vi "SyncVI.vi"(3 "ControlIndicator":T2(array[cluster]), 4 "vi reference":refnum<vi>, 5 "ArrayOfComands":variant) -> (2 "Response":string)   [LabVIEW 2010]
panel:
  out "Temp":string
  out "ArrayOfCommands":T1(array[cluster])
  in  "comand recieved":T3
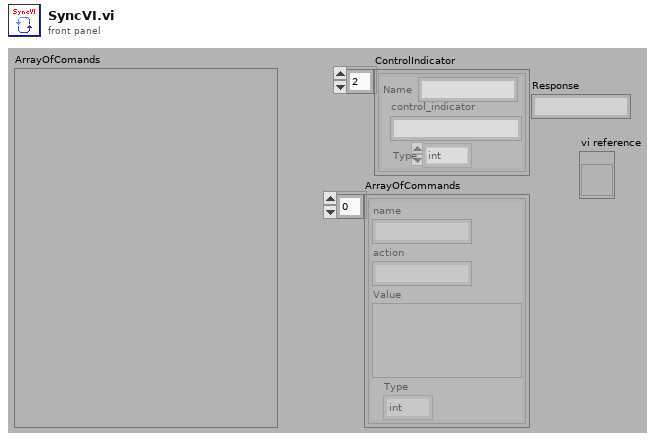
[diagram p1: front panel]
types:
  T1 = cluster{"name":string, "action":string, "Value":variant, "Type":enum16{"int", "boolean", "string", "double", "dateTime", "base64", "struct", "array"}}[]
  T2 = cluster{"Name":string, "control_indicator":string, "Type":enum16{"int", "boolean", "string", "double", "dateTime", "base64", "struct", "array"}}[]
  T3 = cluster{"name":string, "action":string, "Value":variant, "Type":enum16{"int", "boolean", "string", "double", "dateTime", "base64", "struct", "array"}}
  T4 = enum16{"int", "boolean", "string", "double", "dateTime", "base64", "struct", "array"}[]
  T5 = enum16{"int", "boolean", "string", "double", "dateTime", "base64", "struct", "array"}
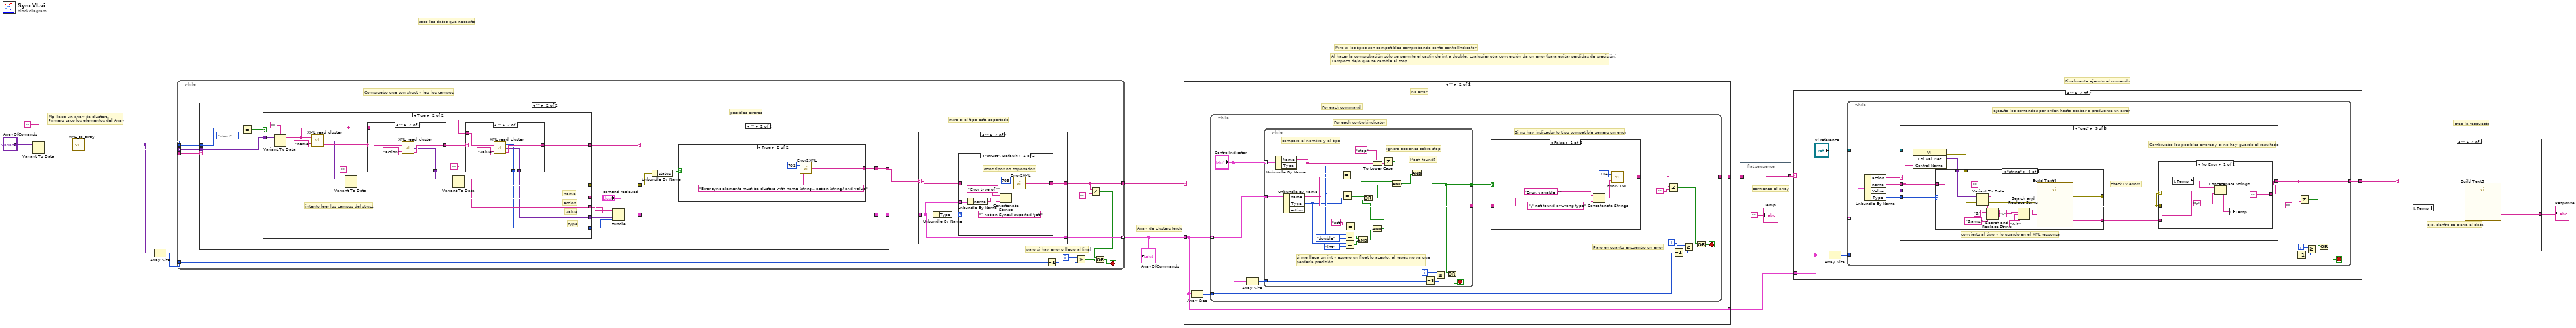
[diagram p0: block diagram]
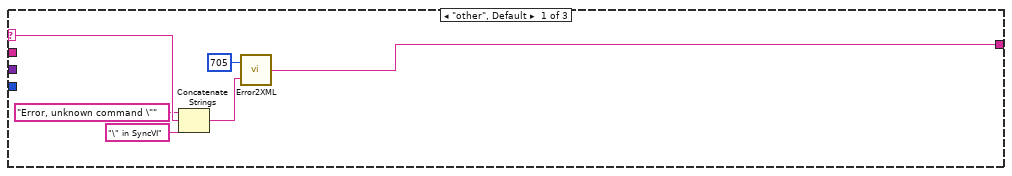
[diagram p4: hidden frame]
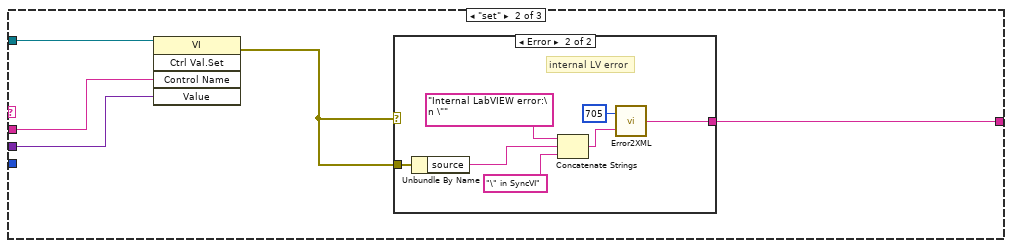
[diagram p5: hidden frame]
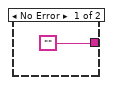
[diagram p6: hidden frame]
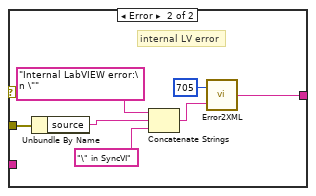
[diagram p7: hidden frame]
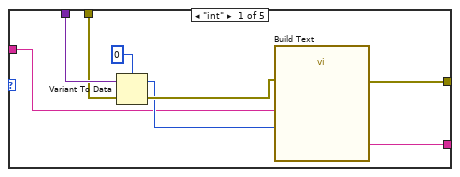
[diagram p8: hidden frame]
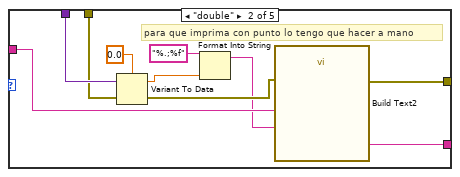
[diagram p9: hidden frame]
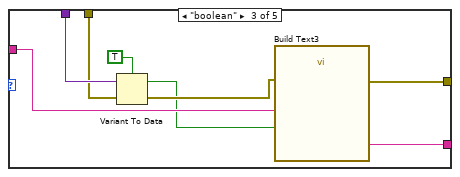
[diagram p10: hidden frame]
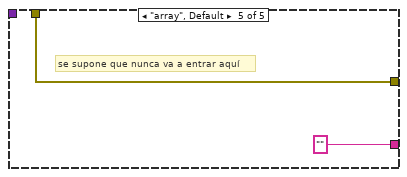
[diagram p11: hidden frame]
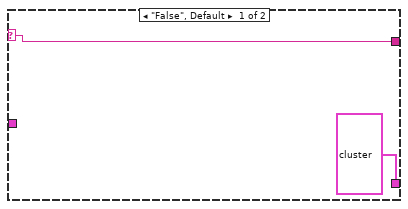
[diagram p12: hidden frame]
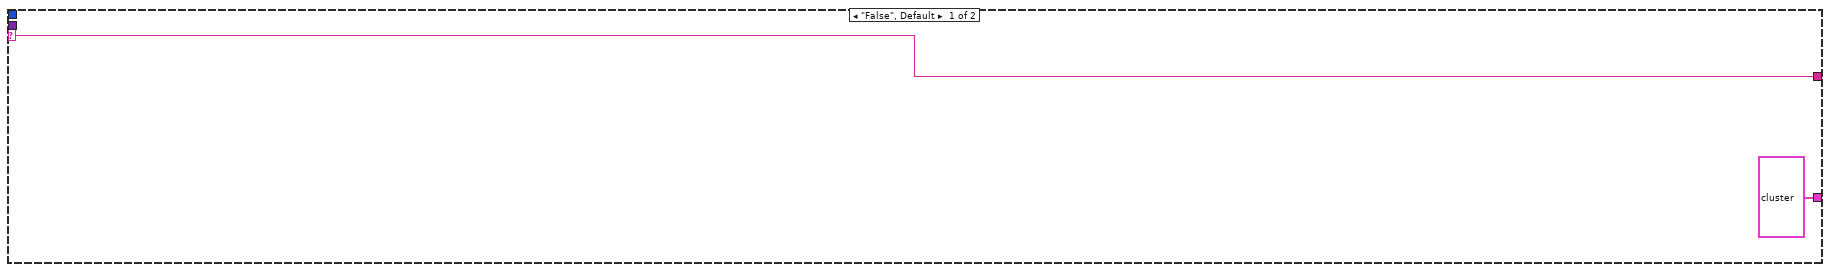
[diagram p14: hidden frame]
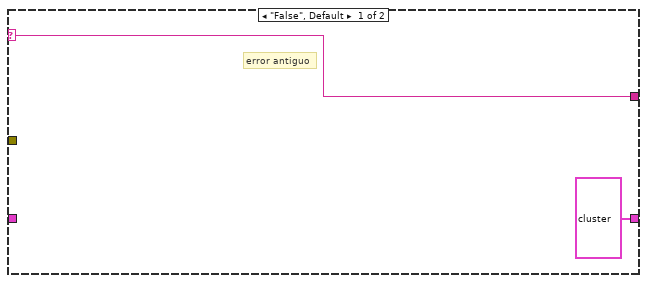
[diagram p15: hidden frame]
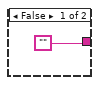
[diagram p16: hidden frame]
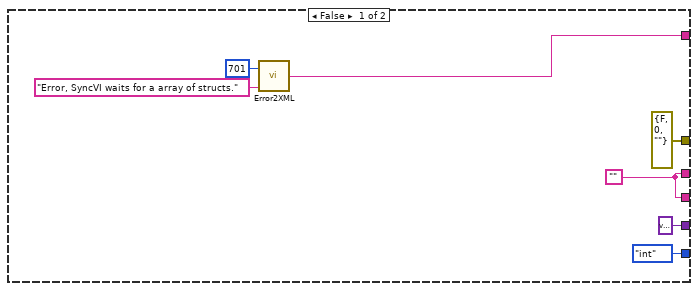
[diagram p17: hidden frame]
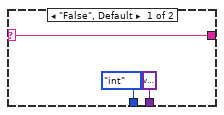
[diagram p18: hidden frame]
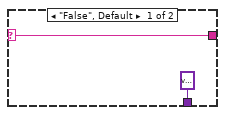
[diagram p19: hidden frame]
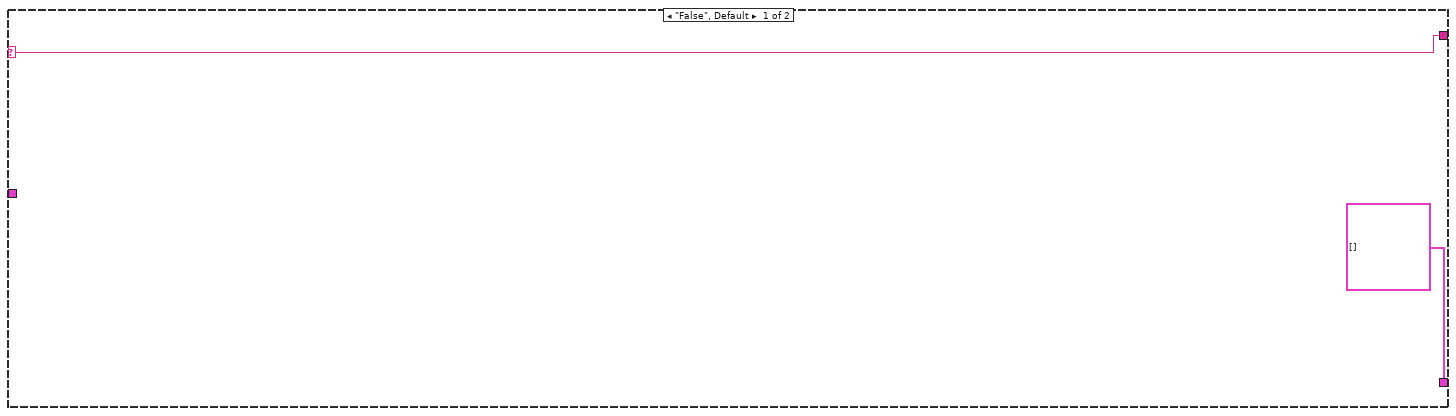
[diagram p20: hidden frame]
diagram:
  # "Al hacer la comprobación sólo se permite el castin de int a double, cualquier otra conversión da un error (para evitar perdidas de precisión)\nTampoco dejo que se cambie el stop"
  # "creo la respuesta"
  # "Finalmente ejecuto el comando"
  # "Miro si los tipos son compatibles comprobando conta controlIndicator"
  # "Array de clusters leido"
  # "saco los datos que necesito"
  # "Me llega un array de clusters.\nPrimero saco los elementos del Array"
  n1 = Variant To Data(Variant="ArrayOfComands", type="") -> (data=w12:string)  [unwired: 1 in, 1 out]
  n2 = call "XML_to_array.vi"("XML"=w12) -> ("ParsingErrors"=w11:string, "Values"=w9:variant[], "Types"=w10:T4)
  n3 = Array Size(array=w9) -> (size(s)=w7:i32)
  n4 = while {
    tunnel: w11 -> [w28]
    tunnel: w10 -> [w27] mode=indexing
    tunnel: w9 -> [w26] mode=indexing
    tunnel: [w17] -> w8
    tunnel: [w23] -> w6 mode=indexing
    tunnel: w7 -> [w21]
    i -> [w22]
    stop <- w19 stop-if-true
    # "paro si hay error o llego al final"
    # "miro si el tipo está soportado"
    # "Compruebo que son struct y leo los campos"
    n5 = case shown="\"\"" w28 {
      selector: w28 -> [w44 _]
      tunnel: w27 -> [_ w58]
      tunnel: w26 -> [_ w55]
      tunnel: [w44 w46] -> w24
      tunnel: [T3 {"name"="", "action"="", "Value"=variant, "Type"=enum."int"} ("comand recieved") w45] -> w25
      frame "False", Default {
      }
      frame "" {
        # "posibles errores"
        n6 = Equal?(x=w58, y=T5."struct") -> (x = y?=w56:bool)
        n7 = case shown="True" w56 {
          tunnel: w55 -> [_ w92]
          tunnel: [w73 w82] -> w54
          tunnel: [errorcluster {"status"=FALSE, "code"=0, "source"=""} ("error out") w79] -> w53
          tunnel: [w71 w81] -> w52
          tunnel: [w71 w80] -> w51
          tunnel: [T5."int" ("Type") w78] -> w49
          tunnel: [variant ("Value") w77] -> w50
          frame False {
            w71 = ""
            n8 = call "Error2XML.vi"("FailDescriptor"="Error, SyncVI waits for a array of structs.", "FailID"=701) -> ("ErrorXML"=w73:string)
          }
          frame True {
            # "type"
            # "value"
            # "action"
            # "name"
            # "intento leer los campos del struct"
            n9 = Variant To Data(Variant=w92, type="") -> (data=w76:string)  [unwired: 1 in, 1 out]
            n10 = call "XML_read_cluster.vi"("Name"="name", "XML"=w76) -> ("ParsingErrors"=w89:string, "Value"=w87:variant)  [unwired: 1 out]
            n11 = Variant To Data(Variant=w87, type="") -> (error out=w85:errorcluster, data=w81:string)  [unwired: 1 in]
            n12 = case shown="\"\"" w89 {
              selector: w89 -> [w102 _]
              tunnel: [w102 w105] -> w88
              tunnel: [variant ("Value") w104] -> w84
              tunnel: w76 -> [_ w103]
              frame "False", Default {
              }
              frame "" {
                n13 = call "XML_read_cluster.vi"("Name"="action", "XML"=w103) -> ("ParsingErrors"=w105:string, "Value"=w104:variant)  [unwired: 1 out]
              }
            }
            n14 = Variant To Data(error in=w85, Variant=w84, type="") -> (error out=w79:errorcluster, data=w80:string)
            n15 = case shown="\"\"" w88 {
              selector: w88 -> [w95 _]
              tunnel: [w95 w100] -> w82
              tunnel: [variant ("Value") w98] -> w77
              tunnel: [T5."int" ("Type") w97] -> w78
              tunnel: w76 -> [_ w96]
              frame "False", Default {
              }
              frame "" {
                n16 = call "XML_read_cluster.vi"("Name"="value", "XML"=w96) -> ("ParsingErrors"=w100:string, "Value"=w98:variant, "Type"=w97:T5)
              }
            }
          }
        }
        n17 = Bundle(cluster="comand recieved", "name"=w52, "action"=w51, "Value"=w50, "Type"=w49) -> (w47:T3)
        n18 = case shown="\"\"" w54 {
          selector: w54 -> [w60 _]
          tunnel: [w60 w64] -> w46
          tunnel: w53 -> [_ w63]
          tunnel: [T3 {"name"="", "action"="", "Value"=variant, "Type"=enum."int"} ("comand recieved") w61] -> w45
          tunnel: w47 -> [_ w61]
          frame "False", Default {
            # "error antiguo"
          }
          frame "" {
            n19 = Unbundle By Name(w63) -> ("status"=w62:bool)
            n20 = case shown="True" w62 {
              tunnel: ["" w66] -> w64
              frame False {
              }
              frame True {
                n21 = call "Error2XML.vi"("FailDescriptor"="Error sync elements must be clusters with name (string), action (string) and value", "FailID"=702) -> ("ErrorXML"=w66:string)
              }
            }
          }
        }
      }
    }
    n22 = case shown="\"\"" w24 {
      selector: w24 -> [w30 w32]
      tunnel: w25 -> [_ w31]
      tunnel: [w30 w33] -> w17
      tunnel: [T3 {"name"="", "action"="", "Value"=variant, "Type"=enum."int"} ("comand recieved") w31] -> w23
      frame "False", Default {
      }
      frame "" {
        n23 = Unbundle By Name(w31) -> ("Type"=w34:T5)
        n24 = case shown="\"struct\", Default" w34 {
          tunnel: w31 -> [w39 _]
          tunnel: [w35 w42] -> w33
          tunnel: w32 -> [_ w42]
          frame "struct", Default {
            # "otros tipos no soportados"
            n25 = Unbundle By Name(w39) -> ("name"=w38:string)
            n26 = Concatenate Strings("Error type of “" ("string"), w38, "” not on SyncVI suported (jet)" ("string")) -> (w40:string)
            n27 = call "Error2XML.vi"("FailDescriptor"=w40, "FailID"=703) -> ("ErrorXML"=w35:string)
          }
          frame "int".."double" {
            # "todo ok"
          }
        }
      }
    }
    n28 = Decrement(x=w21) -> (x-1=w20:i32)
    n29 = Greater Or Equal?(x=w22, y=w20) -> (x >= y?=w18:bool)
    n30 = Not Equal?(x=w17, y="") -> (x != y?=w15:bool)
    n31 = Or(x=w15, y=w18) -> (x .or. y?=w19:bool)
  }
  "ArrayOfCommands" <- w6
  n32 = case shown="\"\"" w8 {
    selector: w8 -> [w108 _]
    tunnel: w6 -> [_ w109]
    tunnel: [w108 w110] -> w4
    tunnel: [T1 [] w109] -> w3
    frame "False", Default {
    }
    frame "" {
      # "no error"
      # "For each command"
      n33 = Array Size(array=w109) -> (size(s)=w111:i32)
      n34 = while {
        tunnel: w109 -> [w119] mode=indexing
        tunnel: w111 -> [w123]
        tunnel: [w114] -> w110
        i -> [w122]
        stop <- w121 stop-if-true
        # "Paro en cuanto encuentro un error"
        # "Si no hay indicador to tipo compatible genero un error"
        # "For each control/indicator"
        n35 = Array Size(array="ControlIndicator") -> (size(s)=w117:i32)
        n36 = while {
          tunnel: "ControlIndicator" -> [w158] mode=indexing
          tunnel: w119 -> [w159]
          tunnel: w117 -> [w155]
          tunnel: [w145] -> w116
          tunnel: [w151] -> w115
          i -> [w154]
          stop <- w153 stop-if-true
          # "si me llega un int y espero un float lo acepto, al revés no ya que \nperdería precisión"
          # "ignoro acciones sobre stop"
          # "Mach found?"
          # "comparo el nombre y el tipo"
          n37 = Unbundle By Name(w158) -> ("Name"=w148:string, "Type"=w142:T5)
          n38 = Unbundle By Name(w159) -> ("name"=w151:string, "Type"=w140:T5, "action"=w136:string)
          n39 = Equal?(x=w148, y=w151) -> (x = y?=w157:bool)
          n40 = Equal?(x=w142, y=w140) -> (x = y?=w144:bool)
          n41 = Equal?(x=w142, y=T5."double") -> (x = y?=w137:bool)
          n42 = Equal?(x=w140, y=T5."int") -> (x = y?=w138:bool)
          n43 = Equal?(x="set", y=w136) -> (x = y?=w132:bool)
          n44 = And(x=w137, y=w138) -> (x .and. y?=w134:bool)
          n45 = And(x=w132, y=w134) -> (x .and. y?=w133:bool)
          n46 = Or(x=w144, y=w133) -> (x .or. y?=w143:bool)
          n47 = To Lower Case(string=w148) -> (all lower case string=w149:string)
          n48 = Not Equal?(x="stop" ("y"), y=w149) -> (x != y?=w147:bool)
          n49 = And(x=w157, y=w143) -> (x .and. y?=w146:bool)
          n50 = And(x=w147, y=w146) -> (x .and. y?=w145:bool)
          n51 = Decrement(x=w155) -> (x-1=w156:i32)
          n52 = Greater Or Equal?(x=w154, y=w156) -> (x >= y?=w152:bool)
          n53 = Or(x=w145, y=w152) -> (x .or. y?=w153:bool)
        }
        n54 = case shown="False" w116 {
          tunnel: w115 -> [w129 _]
          tunnel: [w125 ""] -> w114
          frame False {
            n55 = Concatenate Strings("Error: variable \"", w129, "\" not found or wrong type") -> (w126:string)
            n56 = call "Error2XML.vi"("FailDescriptor"=w126, "FailID"=704) -> ("ErrorXML"=w125:string)
          }
          frame True {
            # "OK"
          }
        }
        n57 = Not Equal?(x=w114, y="") -> (x != y?=w112:bool)
        n58 = Decrement(x=w123) -> (x-1=w124:i32)
        n59 = Greater Or Equal?(x=w122, y=w124) -> (x >= y?=w120:bool)
        n60 = Or(x=w112, y=w120) -> (x .or. y?=w121:bool)
      }
    }
  }
  n61 = flat-sequence {
    tunnel: [w161] -> w5
    tunnel: w4 -> [w161]
    frame #0 {
      # "comienzo el array"
      "Temp" <- ""
    }
  }
  n62 = case shown="\"\"" w5 {
    selector: w5 -> [w162 _]
    tunnel: w3 -> [_ w165]
    tunnel: [w162 w163] -> w2
    frame "False", Default {
    }
    frame "" {
      n63 = Array Size(array=w165) -> (size(s)=w164:i32)
      n64 = while {
        tunnel: "vi reference" -> [w172]
        tunnel: w165 -> [w176] mode=indexing
        tunnel: w164 -> [w177]
        tunnel: [w167] -> w163
        i -> [w168]
        stop <- w178 stop-if-true
        # "ejecuto los comandos por orden hasta acabar o producirse un error"
        n65 = Unbundle By Name(w176) -> ("action"=w175:string, "name"=w174:string, "Value"=w173:variant, "Type"=w171:T5)
        n66 = case shown="\"get\"" w175 {
          selector: w175 -> [w185 _ _]
          tunnel: [w181 w187 w201] -> w167
          tunnel: w174 -> [_ w191 w204]
          tunnel: w173 -> [_ w190 _]
          tunnel: w172 -> [_ w189 w207]
          tunnel: w171 -> [_ _ w206]
          frame "other", Default {
            n67 = Concatenate Strings("Error, unknown command \"" ("string"), w185, "\" in SyncVI" ("string")) -> (w182:string)
            n68 = call "Error2XML.vi"("FailDescriptor"=w182, "FailID"=705) -> ("ErrorXML"=w181:string)
          }
          frame "set" {
            n69 = invoke class="VI" method="Ctrl Val.Set"(reference=w189, "Control Name"=w191, "Value"=w190) -> (error out=w188:errorcluster)  [unwired: 2 in, 4 out]
            n70 = case shown="Error" w188 {
              tunnel: ["" w197] -> w187
              tunnel: w188 -> [_ w194]
              frame No Error {
              }
              frame Error {
                # "internal LV error"
                n71 = Unbundle By Name(w194) -> ("source"=w193:string)
                n72 = Concatenate Strings("Internal LabVIEW error:\n \"" ("string"), w193, "\" in SyncVI" ("string")) -> (w198:string)
                n73 = call "Error2XML.vi"("FailDescriptor"=w198, "FailID"=705) -> ("ErrorXML"=w197:string)
              }
            }
          }
          frame "get" {
            # "Combruebo los posibles errores y si no hay guardo el resultado"
            # "check LV errors"
            # "convierto al tipo y lo guardo en el XML response"
            n74 = invoke class="VI" method="Ctrl Val.Get"(reference=w207, "Control Name"=w204) -> (error out=w203:errorcluster, "Get Control Value Variant"=w205:variant)  [unwired: 2 in, 2 out]
            n75 = case shown="\"string\"" w206 {
              tunnel: w205 -> [w227 w237 w245 w260 _]
              tunnel: [w224 w234 w243 w258 w261] -> w200
              tunnel: w204 -> [w222 w233 w242 w257 _]
              tunnel: [w221 w232 w241 w256 "" ("Result")] -> w202
              tunnel: w203 -> [w220 w231 w238 w246 w261]
              frame "int" {
                n76 = Variant To Data(error in=w220, Variant=w227, type=0) -> (error out=w225:errorcluster, data=w223:i32)
                n77 = call "Build Text"("Name"=w222, "Value"=w223, "error in (no error)"=w225) -> ("Result"=w221:string, "error out"=w224:errorcluster)  [unwired: 11 in]
              }
              frame "double" {
                # "para que imprima con punto lo tengo que hacer a mano"
                n78 = Variant To Data(error in=w231, Variant=w237, type=0.0) -> (error out=w235:errorcluster, data=w229:dbl)
                n79 = Format Into String(format string="%.;%f", w229) -> (resulting string=w228:string)  [unwired: 2 in, 1 out]
                n80 = call "Build Text2"("Name"=w233, "Value"=w228, "error in (no error)"=w235) -> ("Result"=w232:string, "error out"=w234:errorcluster)  [unwired: 11 in]
              }
              frame "boolean" {
                n81 = Variant To Data(error in=w238, Variant=w245, type=TRUE) -> (error out=w244:errorcluster, data=w239:bool)
                n82 = call "Build Text3"("Name"=w242, "Value"=w239, "error in (no error)"=w244) -> ("Result"=w241:string, "error out"=w243:errorcluster)  [unwired: 11 in]
              }
              frame "string" {
                n83 = Variant To Data(error in=w246, Variant=w260, type="") -> (error out=w259:errorcluster, data=w247:string)
                n84 = Search and Replace String(input string=w247, search string="&", replace string="&amp;" ("replace string (\"\")")) -> (result string=w249:string, error out=w250:errorcluster)  [unwired: 5 in, 2 out]
                n85 = Search and Replace String(input string=w249, search string="<", replace string="&lt;" ("replace string (\"\")"), error in=w250) -> (result string=w248:string)  [unwired: 4 in, 3 out]
                n86 = call "Build Text4"("Name"=w257, "Value"=w248, "error in (no error)"=w259) -> ("Result"=w256:string, "error out"=w258:errorcluster)  [unwired: 11 in]
              }
              frame "array", Default {
                # "se supone que nunca va a entrar aquí"
              }
            }
            n87 = case shown="No Error" w200 {
              tunnel: ["" w217] -> w201
              tunnel: w202 -> [w208 _]
              tunnel: w200 -> [_ w213]
              frame No Error {
                n88 = local read "Temp"() -> (w211:string)
                n89 = Concatenate Strings(w211, w208, "\r") -> (w209:string)
                n90 = local write "Temp"(w209) -> ()
              }
              frame Error {
                # "internal LV error"
                n91 = Unbundle By Name(w213) -> ("source"=w214:string)
                n92 = Concatenate Strings("Internal LabVIEW error:\n \"" ("string"), w214, "\" in SyncVI" ("string")) -> (w218:string)
                n93 = call "Error2XML.vi"("FailDescriptor"=w218, "FailID"=705) -> ("ErrorXML"=w217:string)
              }
            }
          }
        }
        n94 = Decrement(x=w177) -> (x-1=w180:i32)
        n95 = Not Equal?(x=w167, y="") -> (x != y?=w169:bool)
        n96 = Greater Or Equal?(x=w168, y=w180) -> (x >= y?=w179:bool)
        n97 = Or(x=w169, y=w179) -> (x .or. y?=w178:bool)
      }
    }
  }
  n98 = case shown="\"\"" w2 {
    selector: w2 -> [w263 _]
    tunnel: [w263 w264] -> w1
    frame "False", Default {
    }
    frame "" {
      # "ojo, dentro se cierra el data"
      n99 = local read "Temp"() -> (w265:string)
      n100 = call "Build Text5"("Temporal data"=w265) -> ("Result"=w264:string)  [unwired: 13 in, 1 out]
    }
  }
  "Response" <- w1
